vi "Sample rate to sample collected.vi"(11 "Sampling Rate _menu":T1(ring)) -> (0 "Sample_rate":u32, 3 "Sample":i32)   [LabVIEW 2017]
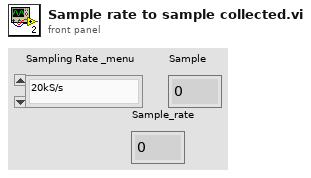
[diagram p1: front panel]
types:
  T1 = enum16{"20kS/s", "10kS/s", "5kS/s", "2kS/s", "1kS/s", "500S/s", "100S/s"}
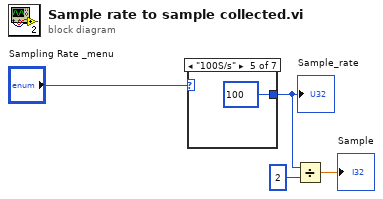
[diagram p0: block diagram]
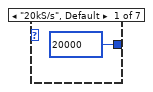
[diagram p2: hidden frame]
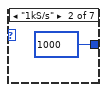
[diagram p3: hidden frame]
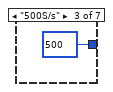
[diagram p4: hidden frame]
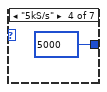
[diagram p5: hidden frame]
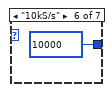
[diagram p6: hidden frame]
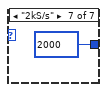
[diagram p7: hidden frame]
diagram:
  n1 = case shown="\"100S/s\"" "Sampling Rate _menu" {
    tunnel: [u32 20000 u32 1000 u32 500 u32 5000 u32 100 u32 10000 u32 2000] -> w1
    frame "20kS/s", Default {
    }
    frame "1kS/s" {
    }
    frame "500S/s" {
    }
    frame "5kS/s" {
    }
    frame "100S/s" {
    }
    frame "10kS/s" {
    }
    frame "2kS/s" {
    }
  }
  "Sample_rate" <- w1
  n2 = Divide(x=w1, y=2) -> (x/y=→"Sample":dbl)
